vi "Get error.vi"(8 "error in (no error)":errorcluster, 11 "Save Image in":refnum<class "Save Image.lvclass">) -> (0 "error out":errorcluster, 2 "error":errorcluster, 3 "Save Image out":refnum<class "Save Image.lvclass">)   [LabVIEW 2018, in "Save Image.lvclass"]
uses:
  Save Image.lvclass
  Save Image.lvclass/Save Image.ctl
  Python Toolkit/Python Toolkit.lvclass
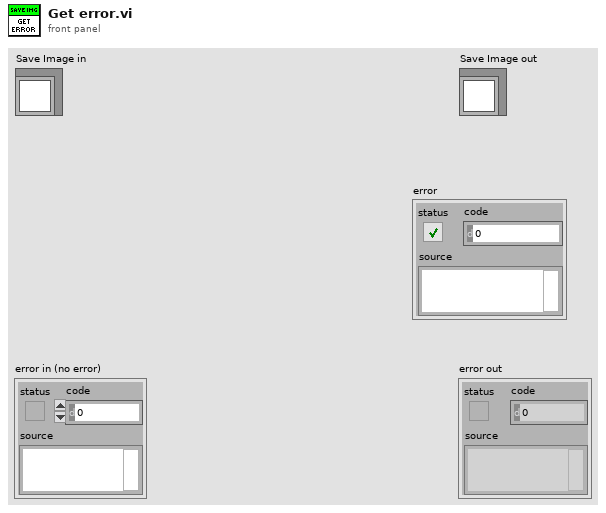
[diagram p1: front panel]
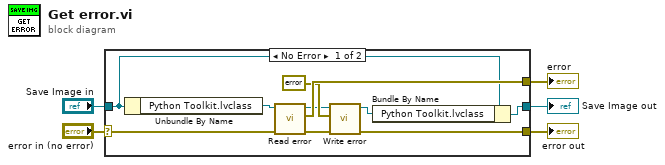
[diagram p0: block diagram]
diagram:
  n1 = case shown="No Error" "error in (no error)" {
    selector: "error in (no error)" -> [w14 w17]
    tunnel: [w12 w17] -> w4
    tunnel: [w8 w16] -> w2
    tunnel: "Save Image in" -> [w9 w16]
    tunnel: [w11 _] -> w1
    frame No Error {
      n2 = Unbundle By Name(w9) -> ("Python Toolkit.lvclass"=w15:refnum<class "Python Toolkit.lvclass">)
      n3 = call-dynamic "Read error.vi"("error in (no error)"=w14, "Python Toolkit in"=w15) -> ("error out"=w13:errorcluster, "error"=w11:errorcluster, "Python Toolkit out"=w6:refnum<class "Python Toolkit.lvclass">)  [unwired: 7 in]
      n4 = call-dynamic "Write error.vi"("error in (no error)"=w13, "error"=errorcluster {"status"=FALSE, "code"=0, "source"=""}, "Python Toolkit in"=w6) -> ("error out"=w12:errorcluster, "Python Toolkit out"=w7:refnum<class "Python Toolkit.lvclass">)  [unwired: 7 in]
      n5 = Bundle By Name(cluster=w9, "Python Toolkit.lvclass"=w7) -> (w8:refnum<class "Save Image.lvclass">)
    }
    frame Error {
    }
  }
  "error out" <- w4
  "Save Image out" <- w2
  "error" <- w1
